vi "Case.vi"   [LabVIEW 2014]
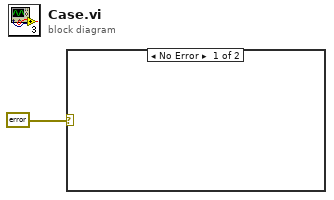
[diagram p0: block diagram]
diagram:
  n1 = case shown="No Error" errorcluster {"status"=FALSE, "code"=0, "source"=""} ("error IO") {
    selector: errorcluster {"status"=FALSE, "code"=0, "source"=""} ("error IO") -> [_ w2]
    frame No Error {
    }
    frame Error {
    }
  }
